vi "Instrument.1820.FloatApprox.vi"(4 "y":dbl, 5 "x":dbl) -> (1 "x ~ y?":bool)   [LabVIEW 2019, in "Instrument.Oxford1820.lvclass"]
doc: "Use to compare floating point numbers. This will check if two numbers are the same to 6 decimal places. Edit block diagram to change tolerance."
uses:
  Instrument.Oxford1820.lvclass
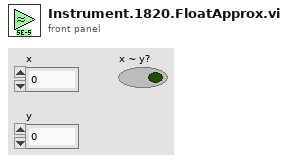
[diagram p1: front panel]
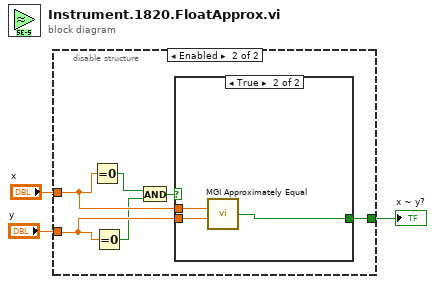
[diagram p0: block diagram]
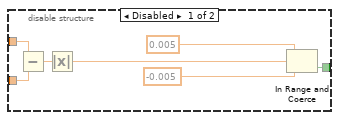
[diagram p2: hidden frame]
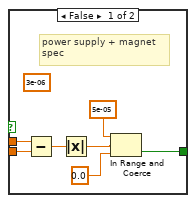
[diagram p3: hidden frame]
diagram:
  n1 = disable-structure shown="Enabled" {
    disable-tunnel: [w10 w16] -> w3
    disable-tunnel: "y" -> [w9 w14]
    disable-tunnel: "x" -> [w8 w15]
    frame Disabled {
      n2 = Subtract(x=w8, y=w9) -> (x-y=w7:dbl)
      n3 = Absolute Value(x=w7) -> (abs(x)=w4:dbl)
      n4 = In Range and Coerce(upper limit=0.005, x=w4, lower limit=-0.005 ("upper limit")) -> (In Range?=w10:bool)  [unwired: 1 out]
    }
    frame Enabled {
      n5 = Equal To 0?(x=w15) -> (x = 0?=w12:bool)
      n6 = Equal To 0?(x=w14) -> (x = 0?=w11:bool)
      n7 = And(x=w12, y=w11) -> (x .and. y?=w13:bool)
      n8 = case shown="True" w13 {
        tunnel: [w23 w25] -> w16
        tunnel: w15 -> [w21 w26]
        tunnel: w14 -> [w22 w24]
        frame False {
          (unwired) 3e-06 ("upper limit")
          # "power supply + magnet\nspec"
          n9 = Subtract(x=w21, y=w22) -> (x-y=w19:dbl)
          n10 = Absolute Value(x=w19) -> (abs(x)=w20:dbl)
          n11 = In Range and Coerce(upper limit=5e-05, x=w20, lower limit=0.0) -> (In Range?=w23:bool)  [unwired: 1 out]
        }
        frame True {
          n12 = call <userlib>:"MGI Approximately Equal.vi"("Numeric 2"=w24, "Numeric 1"=w26) -> ("approx = ?"=w25:bool)
        }
      }
    }
  }
  "x ~ y?" <- w3
